vi "Clear Hardware.vi"(2 "error in (no error)":errorcluster, 3 "Pulseblaster in":refnum<class "Slave_Pulseblaster.lvclass">) -> (0 "error out":errorcluster, 1 "Pulseblaster out":refnum<class "Slave_Pulseblaster.lvclass">)   [LabVIEW 2013, in "Slave_Pulseblaster.lvclass"]
uses:
  Slave_Pulseblaster.lvclass
  Utils_devs/SpinAPI/SpinAPI-Interface.lvlib
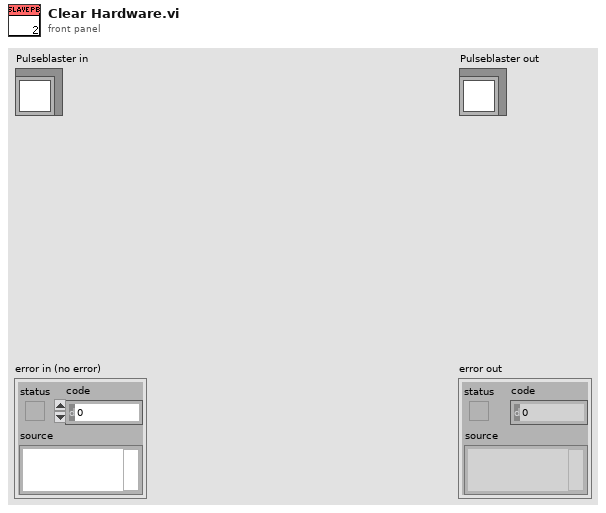
[diagram p1: front panel]
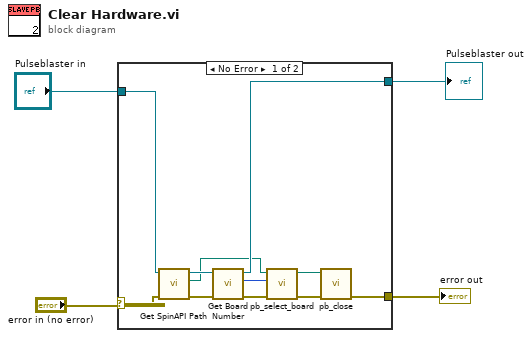
[diagram p0: block diagram]
diagram:
  n1 = case shown="No Error" "error in (no error)" {
    selector: "error in (no error)" -> [w11 w17]
    tunnel: [w10 w17] -> w3
    tunnel: "Pulseblaster in" -> [w13 w16]
    tunnel: [w12 w16] -> w1
    frame No Error {
      n2 = call-dynamic "Get SpinAPI Path.vi"("error in (no error)"=w11, "Pulseblaster in"=w13) -> ("error out"=w15:errorcluster, "SpinAPI Path"=w6:path, "Pulseblaster out"=w14:refnum<class "Slave_Pulseblaster.lvclass">)  [unwired: 7 in]
      n3 = call-dynamic "Get Board Number.vi"("error in (no error)"=w15, "Pulseblaster in"=w14) -> ("error out"=w9:errorcluster, "Board Number"=w5:i32, "Pulseblaster out"=w12:refnum<class "Slave_Pulseblaster.lvclass">)  [unwired: 7 in]
      n4 = call "pb_select_board.vi"("error in (no error)"=w9, "board_num"=w5, "path in"=w6) -> ("error out"=w8:errorcluster, "path out"=w7:path)  [unwired: 7 in]
      n5 = call "pb_close.vi"("error in (no error)"=w8, "path in"=w7) -> ("error out"=w10:errorcluster)  [unwired: 8 in, 1 out]
    }
    frame Error {
    }
  }
  "error out" <- w3
  "Pulseblaster out" <- w1
